vi "Filter Log Packet.vi"(10 "Log Packet":T1, 11 "ILogFilter in":refnum<class "ILogFilter.lvclass">) -> (2 "Log?":bool, 3 "ILogFilter out":refnum<class "ILogFilter.lvclass">)   [LabVIEW 2019, in "Composed Log.lvlib" / "ILogFilter.lvclass"]
uses:
  <vilib>/gpm_packages/@cs/event-logger/Source/Composed Log/ILogFilter/ILogFilter.lvclass
  <vilib>/gpm_packages/@cs/event-logger/Source/Composed Log/Types/Log Packet.ctl
  <vilib>/gpm_packages/@cs/event-logger/Source/Composed Log/Types/Log Level.ctl
  <vilib>/gpm_packages/@cs/event-logger/Source/Composed Log/Composed Log.lvlib
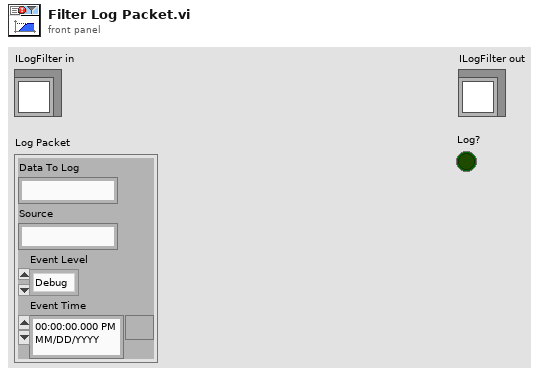
[diagram p1: front panel]
types:
  T1 = typedef "Composed Log.lvlib/Log Packet.ctl" = cluster{"Data To Log":string, "Source":string, "Event Level":T2, "Event Time":timestamp}
  T2 = typedef "Composed Log.lvlib/Log Level.ctl" = enum16{"Debug", "Info", "Warning", "Error", "Critical"}
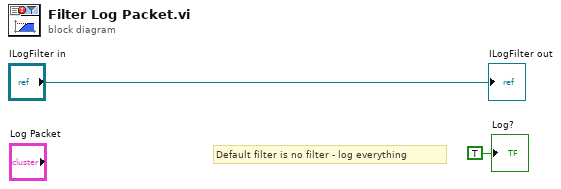
[diagram p0: block diagram]
diagram:
  # "Default filter is no filter - log everything"
  "ILogFilter out" <- "ILogFilter in"
  "Log?" <- TRUE ("Log?")
